vi "_DSF file groups to data.vi"(8 "error in (no error)":errorcluster, 10 "plugin":T3, 11 "configuration file cluster in":T1) -> (0 "error out":errorcluster, 2 "groups":T13[](array[typedef]), 3 "configuration file cluster out":T1)   [LabVIEW 2017, in "DSF Configuration API v1.0.0.lvlib"]
uses:
  DSF Configuration API v1.0.0.lvlib
  Controls/dsf configuration data/1.0.0/dsf settings.ctl
  Controls/dsf configuration data/1.0.0/dsf configuration data v1.0.0.lvlib
  Controls/dsf configuration data/1.0.0/dsf channel.ctl
  Controls/dsf configuration data/1.0.0/dsf transfer.ctl
  Controls/dsf configuration data/1.0.0/dsf timing.ctl
  Controls/dsf configuration data/1.0.0/dsf group.ctl
  get item value by id/get group value by id.vi
  get item value by id/get setting value by id.vi
  Controls/dsf configuration file/1.0.0/dsf timing.ctl
  File API/DSFConfig.lvlib
  Controls/dsf configuration file/1.0.0/DSF Plugin.ctl
  Controls/dsf configuration file/1.0.0/DSF Channel.ctl
  Controls/dsf configuration file/1.0.0/DSF Transfer.ctl
  Controls/dsf configuration file/1.0.0/DSF Group.ctl
  Controls/dsf configuration file/1.0.0/Version Info.ctl
  Controls/dsf configuration file/1.0.0/DSF Settings.ctl
  Controls/dsf configuration file/1.0.0/DSF Config.ctl
  Controls/dsf configuration file/1.0.0/DSF Channel Info.ctl
  Controls/dsf configuration file/1.0.0/DSF Settings Info.ctl
  Controls/dsf configuration file/1.0.0/DSF Transfer Info.ctl
  File API/DSF Plugin Info.ctl
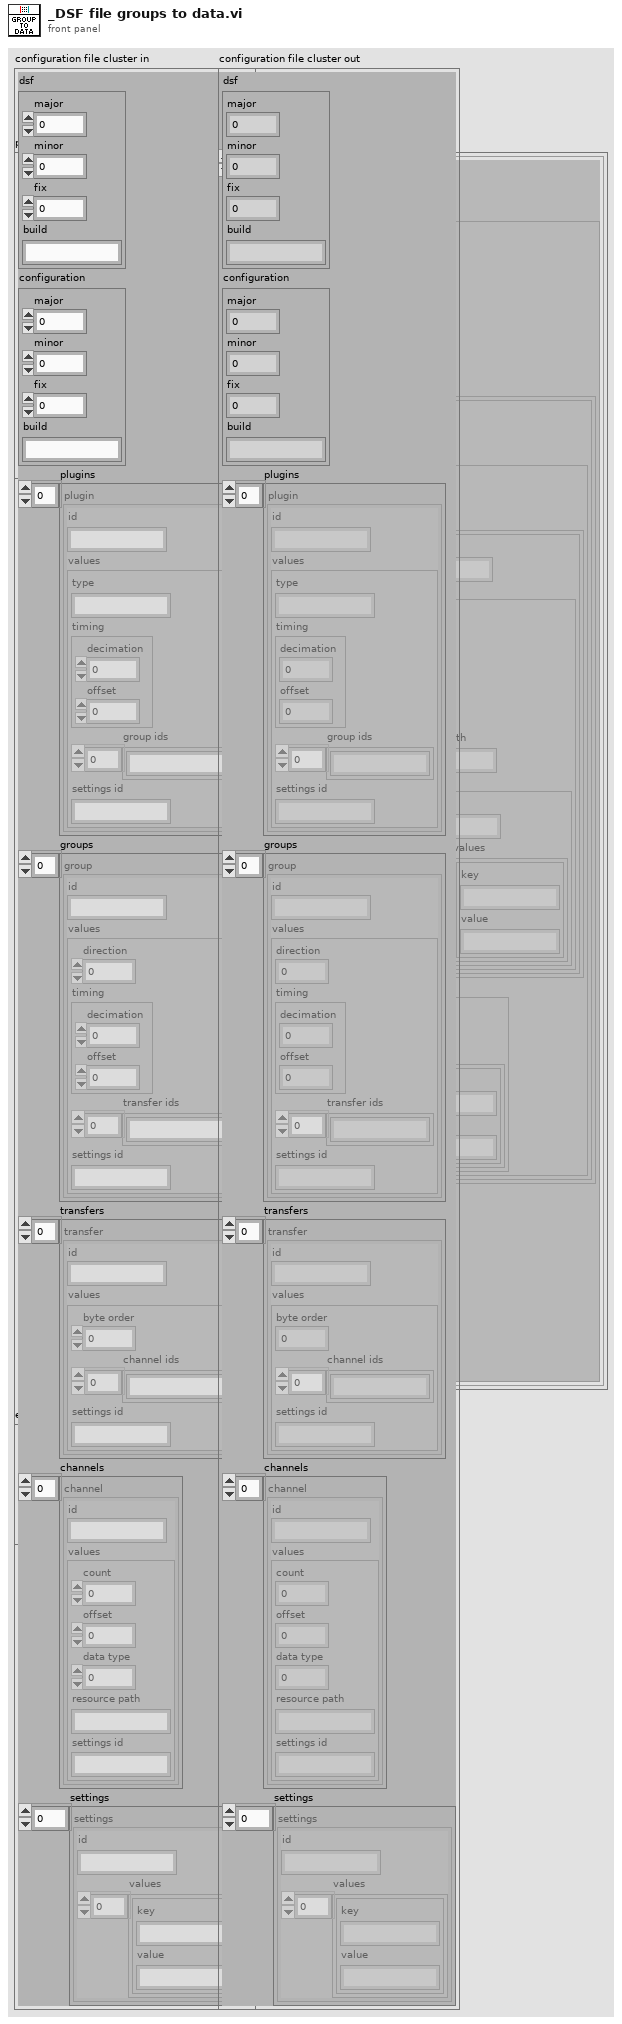
[diagram p1: front panel]
types:
  T1 = typedef "DSFConfig.lvlib/DSF Config.ctl" = cluster{"dsf":T2, "configuration":T2, "plugins":T3[], "groups":T6[], "transfers":T7[], "channels":T9[], "settings":T11[]}
  T2 = typedef "DSFConfig.lvlib/Version Info.ctl" = cluster{"major":u32, "minor":u32, "fix":u32, "build":string}
  T3 = typedef "DSFConfig.lvlib/DSF Plugin.ctl" = cluster{"id":string, "values":T4}
  T4 = typedef "DSFConfig.lvlib/DSF Plugin Info.ctl" = cluster{"type":string, "timing":T5, "group ids":string[], "settings id":string}
  T5 = typedef "DSFConfig.lvlib/dsf timing.ctl" = cluster{"decimation":i32, "offset":i32}
  T6 = typedef "DSFConfig.lvlib/DSF Group.ctl" = cluster{"id":string, "values":cluster{"direction":i32, "timing":T5, "transfer ids":string[], "settings id":string}}
  T7 = typedef "DSFConfig.lvlib/DSF Transfer.ctl" = cluster{"id":string, "values":T8}
  T8 = typedef "DSFConfig.lvlib/DSF Transfer Info.ctl" = cluster{"byte order":i32, "channel ids":string[], "settings id":string}
  T9 = typedef "DSFConfig.lvlib/DSF Channel.ctl" = cluster{"id":string, "values":T10}
  T10 = typedef "DSFConfig.lvlib/DSF Channel Info.ctl" = cluster{"count":i32, "offset":i32, "data type":i32, "resource path":string, "settings id":string}
  T11 = typedef "DSFConfig.lvlib/DSF Settings.ctl" = cluster{"id":string, "values":T12}
  T12 = typedef "DSFConfig.lvlib/DSF Settings Info.ctl" = cluster{"key":string, "value":string}[]
  T13 = typedef "dsf configuration data v1.0.0.lvlib/dsf group.ctl" = cluster{"id":string, "values":cluster{"direction":i32, "timing":T14, "transfers":T15[], "settings":T17}}
  T14 = typedef "dsf configuration data v1.0.0.lvlib/dsf timing.ctl" = cluster{"decimation":i32, "offset":i32}
  T15 = typedef "dsf configuration data v1.0.0.lvlib/dsf transfer.ctl" = cluster{"id":string, "values":cluster{"byte order":i32, "channels":T16[], "settings":T17}}
  T16 = typedef "dsf configuration data v1.0.0.lvlib/dsf channel.ctl" = cluster{"id":string, "values":cluster{"count":i32, "offset":i32, "data type":i32, "resource path":string, "settings":T17}}
  T17 = typedef "dsf configuration data v1.0.0.lvlib/dsf settings.ctl" = cluster{"id":string, "values":cluster{"key":string, "value":string}[]}
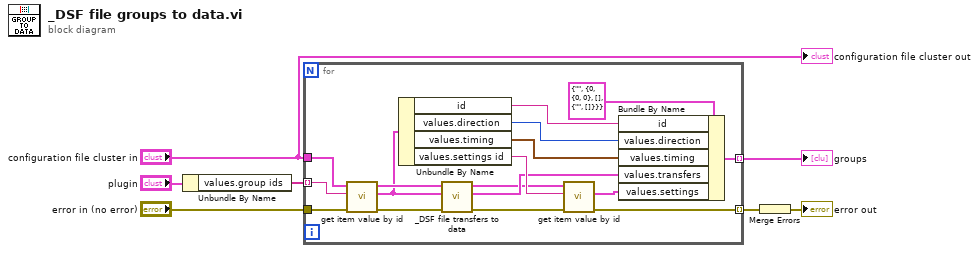
[diagram p0: block diagram]
diagram:
  n1 = Unbundle By Name("plugin") -> ("values.group ids"=w3:string[])
  n2 = for {
    tunnel: w3 -> [w24] mode=indexing
    tunnel: "configuration file cluster in" -> [w23]
    tunnel: [w18] -> w1 mode=indexing
    tunnel: "error in (no error)" -> [w14]
    tunnel: [w11] -> w6 mode=indexing
    n3 = call-poly "get item value by id.vi"("error in (no error)"=w14, "id"=w24, "configuration file cluster in"=w23) -> ("error out"=w13:errorcluster, "group"=w10:T6, "configuration file cluster out"=w17:T1)  [unwired: 5 in, 1 out]
    n4 = Unbundle By Name(w10) -> ("id"=w21:string, "values.direction"=w20:i32, "values.timing"=w19:T5, "values.settings id"=w16:string)
    n5 = call "_DSF file transfers to data.vi"("error in (no error)"=w13, "group"=w10, "configuration file cluster in"=w17) -> ("error out"=w12:errorcluster, "transfers"=w9:T15[], "configuration file cluster out"=w8:T1)  [unwired: 6 in]
    n6 = call-poly "get item value by id.vi"("error in (no error)"=w12, "id"=w16, "configuration file cluster in"=w8) -> ("error out"=w11:errorcluster, "settings"=w15:T11)  [unwired: 5 in, 2 out]
    n7 = Bundle By Name(cluster=T13 {"id"="", "values"={"direction"=0, "timing"={"decimation"=0, "offset"=0}, "transfers"=[], "settings"={"id"="", "values"=[]}}} ("group"), "id"=w21, "values.direction"=w20, "values.timing"=w19, "values.transfers"=w9, "values.settings"=w15) -> (w18:T13)
  }
  "groups" <- w1
  n8 = Merge Errors(w6) -> (→"error out":errorcluster)
  "configuration file cluster out" <- "configuration file cluster in"
